vi "Get-Set-Ctrl-Indi-Value.vi"(0 "Quick-GUI-Update in":refnum<class "Quick-GUI-Update.lvclass">, 2 "Lable":string, 7 "Value In":variant, 11 "error in (no error)":errorcluster, 13 "Set-Value?":bool) -> (4 "Quick-GUI-Update out":refnum<class "Quick-GUI-Update.lvclass">, 6 "Specified Ctrl Ref":refnum<vi>[](array[refnum]), 8 "Value Out":variant, 10 "Not Empty Value?":bool, 15 "error IO":errorcluster)   [LabVIEW 2020, in "Quick-GUI-Update.lvclass"]
uses:
  Quick-GUI-Update.lvclass
  Quick-GUI-Update.lvclass/Quick-GUI-Update.ctl
  Ctrl Reference's/Ctrl Reference's.lvclass
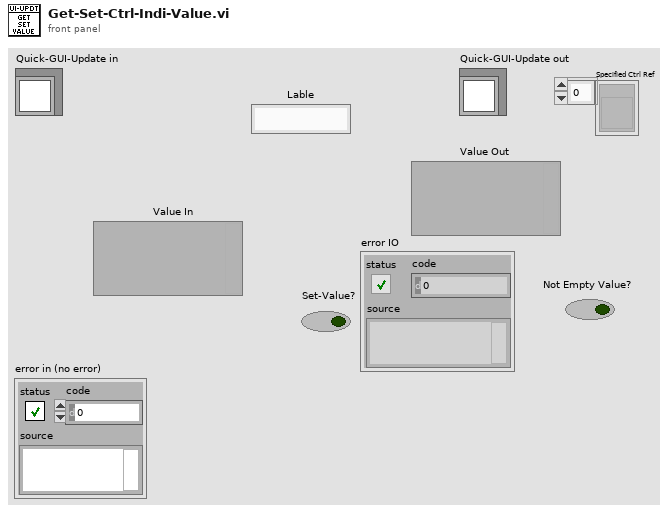
[diagram p1: front panel]
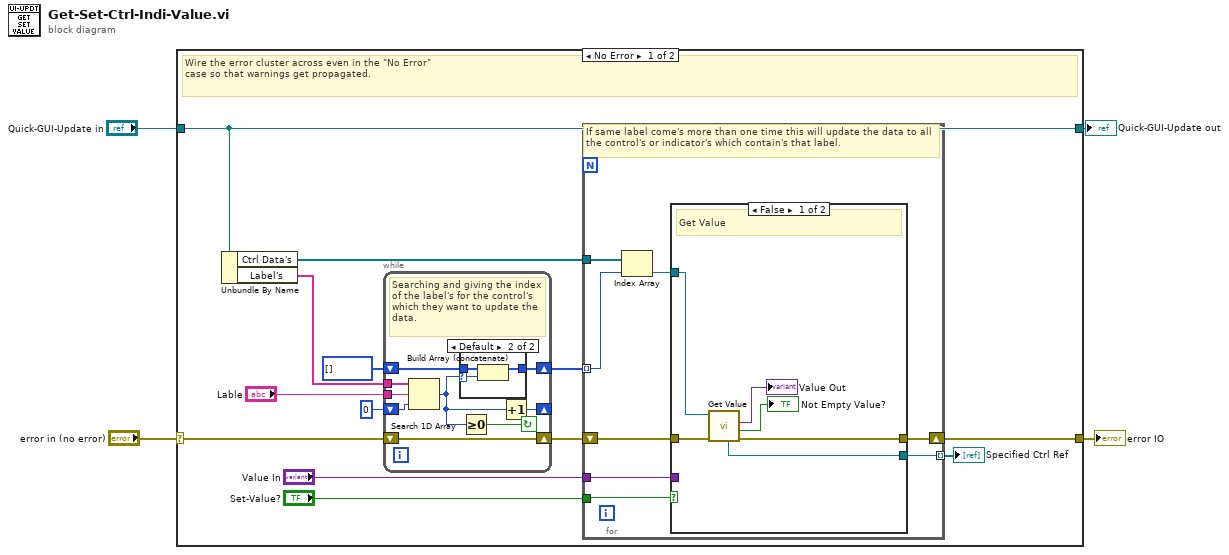
[diagram p0: block diagram]
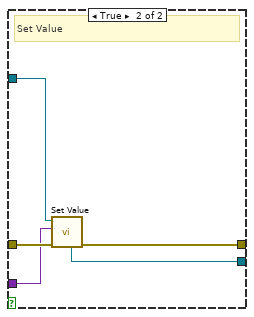
[diagram p3: hidden frame]
diagram:
  n1 = case shown="No Error" "error in (no error)" {
    selector: "error in (no error)" -> [w12 w50]
    tunnel: [w8 w51] -> w2
    tunnel: "Quick-GUI-Update in" -> [w8 w51]
    tunnel: [w7 w50] -> w1
    frame No Error {
      # "Wire the error cluster across even in the \"No Error\"\ncase so that warnings get propagated."
      n2 = Unbundle By Name(w8) -> ("Ctrl Data's"=w6:refnum<class "Ctrl Reference's.lvclass">[], "Label's"=w9:string[])
      n3 = while {
        shift-right: [w20] -> _
        shift-left: 0 ("Start Index (0)") -> [w26]
        shift-right: [w24] -> w15
        shift-left: i32[] [] ("Initial Elements") -> [w25]
        tunnel: "Lable" -> [w23]
        shift-right: [w19] -> w14
        shift-left: w12 -> [w19]
        tunnel: w9 -> [w18]
        stop <- w21 continue-if-true
        # "Searching and giving the index of the label's for the control's which they want to update the data."
        n4 = Search 1D Array(1D array=w18, element=w23, start index (0)=w26) -> (index of element=w22:i32)
        n5 = case shown="Default" w22 {
          selector: w22 -> [_ w30]
          tunnel: w25 -> [w27 w29]
          tunnel: [w27 w28] -> w24
          frame -1 {
          }
          frame Default {
            n6 = Build Array (concatenate)(w29, w30) -> (w28:i32[])
          }
        }
        n7 = Greater Or Equal To 0?(x=w22) -> (x >= 0?=w21:bool)
        n8 = Increment(x=w22) -> (x+1=w20:i32)
      }
      n9 = for {
        tunnel: "Set-Value?" -> [w38]
        shift-right: [w37] -> w7
        shift-left: w14 -> [w32]
        tunnel: w15 -> [w35] mode=indexing
        tunnel: "Value In" -> [w34]
        tunnel: w6 -> [w36]
        tunnel: [w31] -> w5 mode=indexing
        # "If same label come's more than one time this will update the data to all the control's or indicator's which contain's that label."
        n10 = Index Array(array=w36, index=w35) -> (element=w33:refnum<class "Ctrl Reference's.lvclass">)
        n11 = case shown="False" w38 {
          tunnel: [w41 w46] -> w37
          tunnel: w32 -> [w42 w49]
          tunnel: w34 -> [_ w48]
          tunnel: w33 -> [w44 w47]
          tunnel: [w39 w45] -> w31
          frame False {
            # "Get Value"
            n12 = call "Get Value.vi"("error in (no error)"=w42, "Ctrl Reference's in"=w44) -> ("error out"=w41:errorcluster, "Not Empty Value?"=→"Not Empty Value?":bool, "Value Out"=→"Value Out":variant, "Ctl Refnum"=w39:refnum<vi>)  [unwired: 5 in, 1 out]
          }
          frame True {
            # "Set Value"
            n13 = call "Set Value.vi"("error in (no error)"=w49, "Value"=w48, "Ctrl Reference's in"=w47) -> ("error out"=w46:errorcluster, "Ctl Refnum"=w45:refnum<vi>)  [unwired: 6 in, 1 out]
          }
        }
      }
      "Specified Ctrl Ref" <- w5
    }
    frame Error {
    }
  }
  "Quick-GUI-Update out" <- w2
  "error IO" <- w1
